vi "DC Bias Level.vi"(7 "Level Selector (T: Volt)":bool=TRUE, 8 "error in (no error)":errorcluster, 9 "Current Level (A) (0.0)":dbl min=-0.1 max=1.0 step=0.001 format="%.4f", 10 "Voltage Level (V) (0.0)":dbl min=-40.0 max=40.0 step=0.1 format="%.4f", 11 "VISA resource name":refnum<visa-resource-name>) -> (0 "error out":errorcluster, 3 "VISA resource name out":refnum<visa-resource-name>)   [LabVIEW 2015, in "Agilent 428X Series.lvlib"]
doc: "The Bias Level function sets the DC bias Voltage/Current. Setting bias voltage/current does not implicitly turn the DC bias ON. This function is effective when the Option 001 Bias is installed or the HP 42841A and the HP 42842C are combine."
uses:
  <instrlib>/Agilent 428X Series/Agilent 428X Series.lvlib
panel:
  # "Voltage\nCurrent"
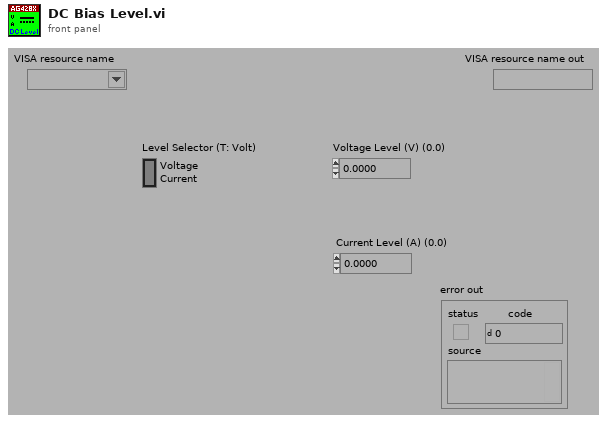
[diagram p1: front panel]
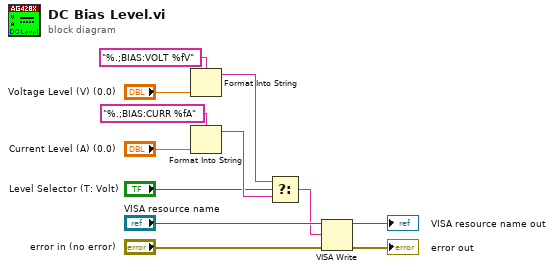
[diagram p0: block diagram]
diagram:
  n1 = Format Into String(format string="%.;BIAS:VOLT %fV", "Voltage Level (V) (0.0)") -> (resulting string=w3:string)  [unwired: 2 in, 1 out]
  n2 = Format Into String(format string="%.;BIAS:CURR %fA", "Current Level (A) (0.0)") -> (resulting string=w2:string)  [unwired: 2 in, 1 out]
  n3 = Select(t=w3, s="Level Selector (T: Volt)", f=w2) -> (s? t:f=w4:string)
  n4 = VISA Write(VISA resource name="VISA resource name", write buffer=w4, error in (no error)="error in (no error)") -> (VISA resource name out=→"VISA resource name out":refnum<visa-resource-name>, error out=→"error out":errorcluster)  [unwired: 1 out]
